vi "GDSII Playground.vi"() -> ()   [LabVIEW 2020]
uses:
  Record/Record.lvclass
panel:
  out "Array 2":string[](array[string])
  out "size(s)":i32
  out "Array":string[](array[string])
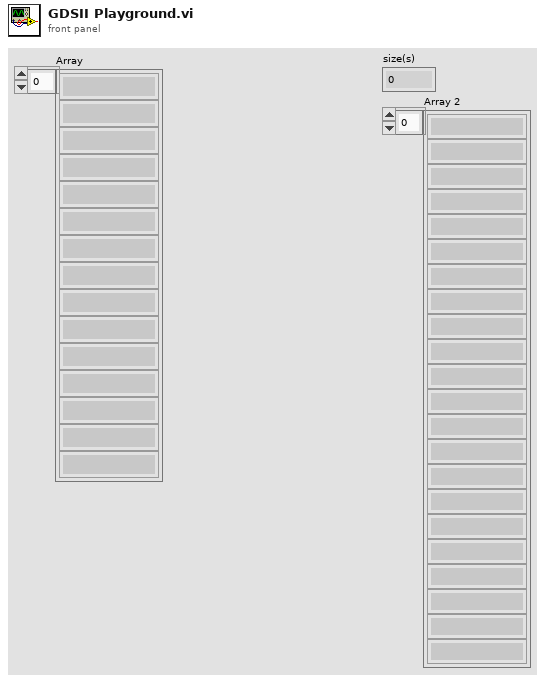
[diagram p1: front panel]
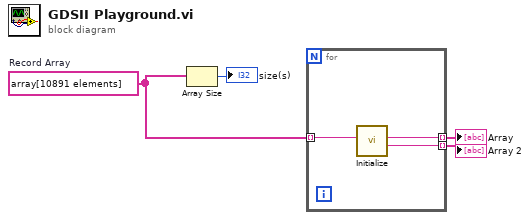
[diagram p0: block diagram]
diagram:
  w3 = string[] array[10891 elements]  # Record Array
  n1 = Array Size(array=w3) -> (size(s)=→"size(s)":i32)
  n2 = for {
    tunnel: w3 -> [w7] mode=indexing
    tunnel: [w6] -> w4 mode=indexing
    tunnel: [w5] -> w1 mode=indexing
    n3 = call "Initialize.vi"("Raw Record String"=w7) -> ("value 2"=w5:string, "value"=w6:string)  [unwired: 7 in, 2 out]
  }
  "Array" <- w4
  "Array 2" <- w1
